vi "ScaleRawData.vi"(4 "Vx,Vy,Vsum as signals or\ntrue X,Y,Z signal (1,default)":bool=TRUE, 5 "error in (no error)":errorcluster, 6 "All DAQ channels":T3, 7 "Scale Option":i32(ring)=2 items=["ScaleButDoNotCalculatePsi", "CalculatePsi, ButDoNotCompensate", "CompensationAllSignalsByCalcuatedPsi", "DoNotScale(ReadRawVoltageSignals)"], 8 "Params in":T8={"Manual Control"={"Rotation Control"={"Phase"=0.0, "A amp (0-120)"=75.0, "B amp (0-120)"=53.3, "mean freq  [MHz]\ndefault 39.99"=40.0, "freq difference [Hz]"=2.0, "Enable A"=TRUE, "Enable B"=TRUE}, "X piezo\n [nm]"=0.0, "Y peizo\n [nm]"=0.0, "-Z piezo\n [nm]"=5.012658227848101, "AOM0 \nPower"=0.2}, "Piezo Calibr"={"Px2Vx(AO)"=nan, "Py2Vy(AO)"=nan, "Pz2Vz(AO)"=nan, "Min Px"=nan, "Min Py"=nan, "Min Pz"=nan, "Max Px"=nan, "Max Py"=nan, "Max Pz"=nan}, "Instrument Calibr"={"TQGT"=[], "TetherCenter"={"TrapX_AO 0 [nm]"=nan, "TrapY_AO 0 [nm]"=nan, "TrapZ_AO 0 [nm]"=nan}, "XYZsignal baseline"={"Xsignal0"=nan, "Ysignal0"=nan, "Zsignal0"=nan, "Zsig slope"=nan, "Z bead0"=nan}, "S and P to Vs0"={"Vs0/P"=1.0, "Vs0/S"=1.0}, "Psi"=0.0, "ePS:eRL drift correlation"={"Interc P"=nan, "Slope P"=nan, "Interc S"=nan, "Slope S"=nan}, "Current piezo volt AO"={"Vpx_AO [V]"=nan, "Vpy_AO [V]"=nan, "Vpz_AO [V]"=nan}}, "Cylinder Calibr"={"ZStiff"=nan, "Zsens"=nan, "AngStiff"=nan, "XStiff"=nan, "Xsens"=nan, "MaxEllip"=nan, "YStiff"=nan, "Ysens"=nan, "FocalShift"=nan, "Sfz"=nan, "1/Sz"=nan, "Stau"=nan, "Sfx"=nan, "1/Sx"=nan, "1/Sang"=nan, "Sfy"=nan, "1/Sy"=nan, "1/focal"=nan}, "DAQParams"={"Buffer size"=nan, "Scanning rate"=nan, "Average"=nan, "Sampling rate"=nan, "set dt"=nan}, "DAQ channel offsets"={"A0 [V]"=0.0, "D0 [V]"=0.0, "P0  [V]"=0.0, "S0 [V]"=0.0, "L0 [V]"=0.0, "R0 [V]"=0.0, "Vpx0 [V]"=0.0, "Vpy0 [V]"=0.0, "Vpz0 [V]"=0.0, "Vsum0 [V]"=0.0, "Vpx_AO0 [V]"=0.0, "Vpy_AO0 [V]"=0.0, "Vpz_AO0 [V]"=0.0}, "Z bead polynomial coeffs"=[nan, nan, nan, nan], "Skip button ref"=refnum, "z bead lookup table"={"z signal"=[], "z bead"=[]}, "SP->power Matrix"=[], "Ms2p"=[], "Mp2s"=[], "task in"="Oscilloscope2"} {"Instrument Calibr"."Psi" format="%#_2f"; "Manual Control"."Y peizo\n [nm]" scale=0.0..7000.0; "Manual Control"."AOM0 \nPower" scale=0.0..1.0; "Manual Control"."X piezo\n [nm]" scale=0.0..7000.0; "Manual Control"."Rotation Control"."freq difference [Hz]" step=0.5; "Manual Control"."Rotation Control"."mean freq  [MHz]\ndefault 39.99" min=0.0 step=0.01; "Manual Control"."Rotation Control"."B amp (0-120)" min=0.0 max=120.0 step=0.1; "Manual Control"."Rotation Control"."A amp (0-120)" min=0.0 max=120.0 step=0.1; "Manual Control"."Rotation Control"."Phase" scale=0.0..360.0; "Manual Control"."-Z piezo\n [nm]" scale=1000.0..7000.0}) -> (0 "error out":errorcluster, 1 "Scaled data":T7, 2 "All DAQ channels out":T3, 3 "Params out":T8={"Manual Control"={"Rotation Control"={"Phase"=0.0, "A amp (0-120)"=75.0, "B amp (0-120)"=53.3, "mean freq  [MHz]\ndefault 39.99"=40.0, "freq difference [Hz]"=2.0, "Enable A"=TRUE, "Enable B"=TRUE}, "X piezo\n [nm]"=0.0, "Y peizo\n [nm]"=0.0, "-Z piezo\n [nm]"=5.012658227848101, "AOM0 \nPower"=0.2}, "Piezo Calibr"={"Px2Vx(AO)"=nan, "Py2Vy(AO)"=nan, "Pz2Vz(AO)"=nan, "Min Px"=nan, "Min Py"=nan, "Min Pz"=nan, "Max Px"=nan, "Max Py"=nan, "Max Pz"=nan}, "Instrument Calibr"={"TQGT"=[], "TetherCenter"={"TrapX_AO 0 [nm]"=nan, "TrapY_AO 0 [nm]"=nan, "TrapZ_AO 0 [nm]"=nan}, "XYZsignal baseline"={"Xsignal0"=nan, "Ysignal0"=nan, "Zsignal0"=nan, "Zsig slope"=nan, "Z bead0"=nan}, "S and P to Vs0"={"Vs0/P"=1.0, "Vs0/S"=1.0}, "Psi"=0.0, "ePS:eRL drift correlation"={"Interc P"=nan, "Slope P"=nan, "Interc S"=nan, "Slope S"=nan}, "Current piezo volt AO"={"Vpx_AO [V]"=nan, "Vpy_AO [V]"=nan, "Vpz_AO [V]"=nan}}, "Cylinder Calibr"={"ZStiff"=nan, "Zsens"=nan, "AngStiff"=nan, "XStiff"=nan, "Xsens"=nan, "MaxEllip"=nan, "YStiff"=nan, "Ysens"=nan, "FocalShift"=nan, "Sfz"=nan, "1/Sz"=nan, "Stau"=nan, "Sfx"=nan, "1/Sx"=nan, "1/Sang"=nan, "Sfy"=nan, "1/Sy"=nan, "1/focal"=nan}, "DAQParams"={"Buffer size"=nan, "Scanning rate"=nan, "Average"=nan, "Sampling rate"=nan, "set dt"=nan}, "DAQ channel offsets"={"A0 [V]"=0.0, "D0 [V]"=0.0, "P0  [V]"=0.0, "S0 [V]"=0.0, "L0 [V]"=0.0, "R0 [V]"=0.0, "Vpx0 [V]"=0.0, "Vpy0 [V]"=0.0, "Vpz0 [V]"=0.0, "Vsum0 [V]"=0.0, "Vpx_AO0 [V]"=0.0, "Vpy_AO0 [V]"=0.0, "Vpz_AO0 [V]"=0.0}, "Z bead polynomial coeffs"=[nan, nan, nan, nan], "Skip button ref"=refnum, "z bead lookup table"={"z signal"=[], "z bead"=[]}, "SP->power Matrix"=[], "Ms2p"=[], "Mp2s"=[], "task in"="Oscilloscope2"} {"Instrument Calibr"."Psi" format="%#_2f"; "Manual Control"."Y peizo\n [nm]" scale=0.0..7000.0; "Manual Control"."AOM0 \nPower" scale=0.0..1.0; "Manual Control"."X piezo\n [nm]" scale=0.0..7000.0; "Manual Control"."Rotation Control"."freq difference [Hz]" step=0.5; "Manual Control"."Rotation Control"."mean freq  [MHz]\ndefault 39.99" min=0.0 step=0.01; "Manual Control"."Rotation Control"."B amp (0-120)" min=0.0 max=120.0 step=0.1; "Manual Control"."Rotation Control"."A amp (0-120)" min=0.0 max=120.0 step=0.1; "Manual Control"."Rotation Control"."Phase" scale=0.0..360.0; "Manual Control"."-Z piezo\n [nm]" scale=1000.0..7000.0})   [LabVIEW 2017, in "SignalConverson.lvlib"]
uses:
  SignalConverson.lvlib
  <vilib>/Analysis/NI_AALBase.lvlib
  <vilib>/Analysis/baseanly.llb/A x Vector.vi
  Angle compensated data.ctl
  XYZ Signals.ctl
  Measrured TrapXYZ.ctl
  Set TrapXYZ.ctl
  Data Before Angle Compensation.ctl
  Initialization/Param.ctl
  Initialization/ManualCtrl.ctl
  Initialization/Initialization.lvlib
  Initialization/CylinderCalibrNew.ctl
  <vilib>/Analysis/Matrix/Datatypes/RealMatrix.ctl
  <vilib>/Analysis/Matrix/NI_Matrix.lvlib
  DAQChannelRawData.ctl
  DAQChannelOffsets.ctl
  ScaledData.ctl
panel:
  out "Data before TCT":T1
  out "set TrapXYZ":T2
  out "Measured Piezo Position":T4
  out "X,Y,Z signal":T5
  out "Data after TCT":T6
  out "Data Before TCT":T1
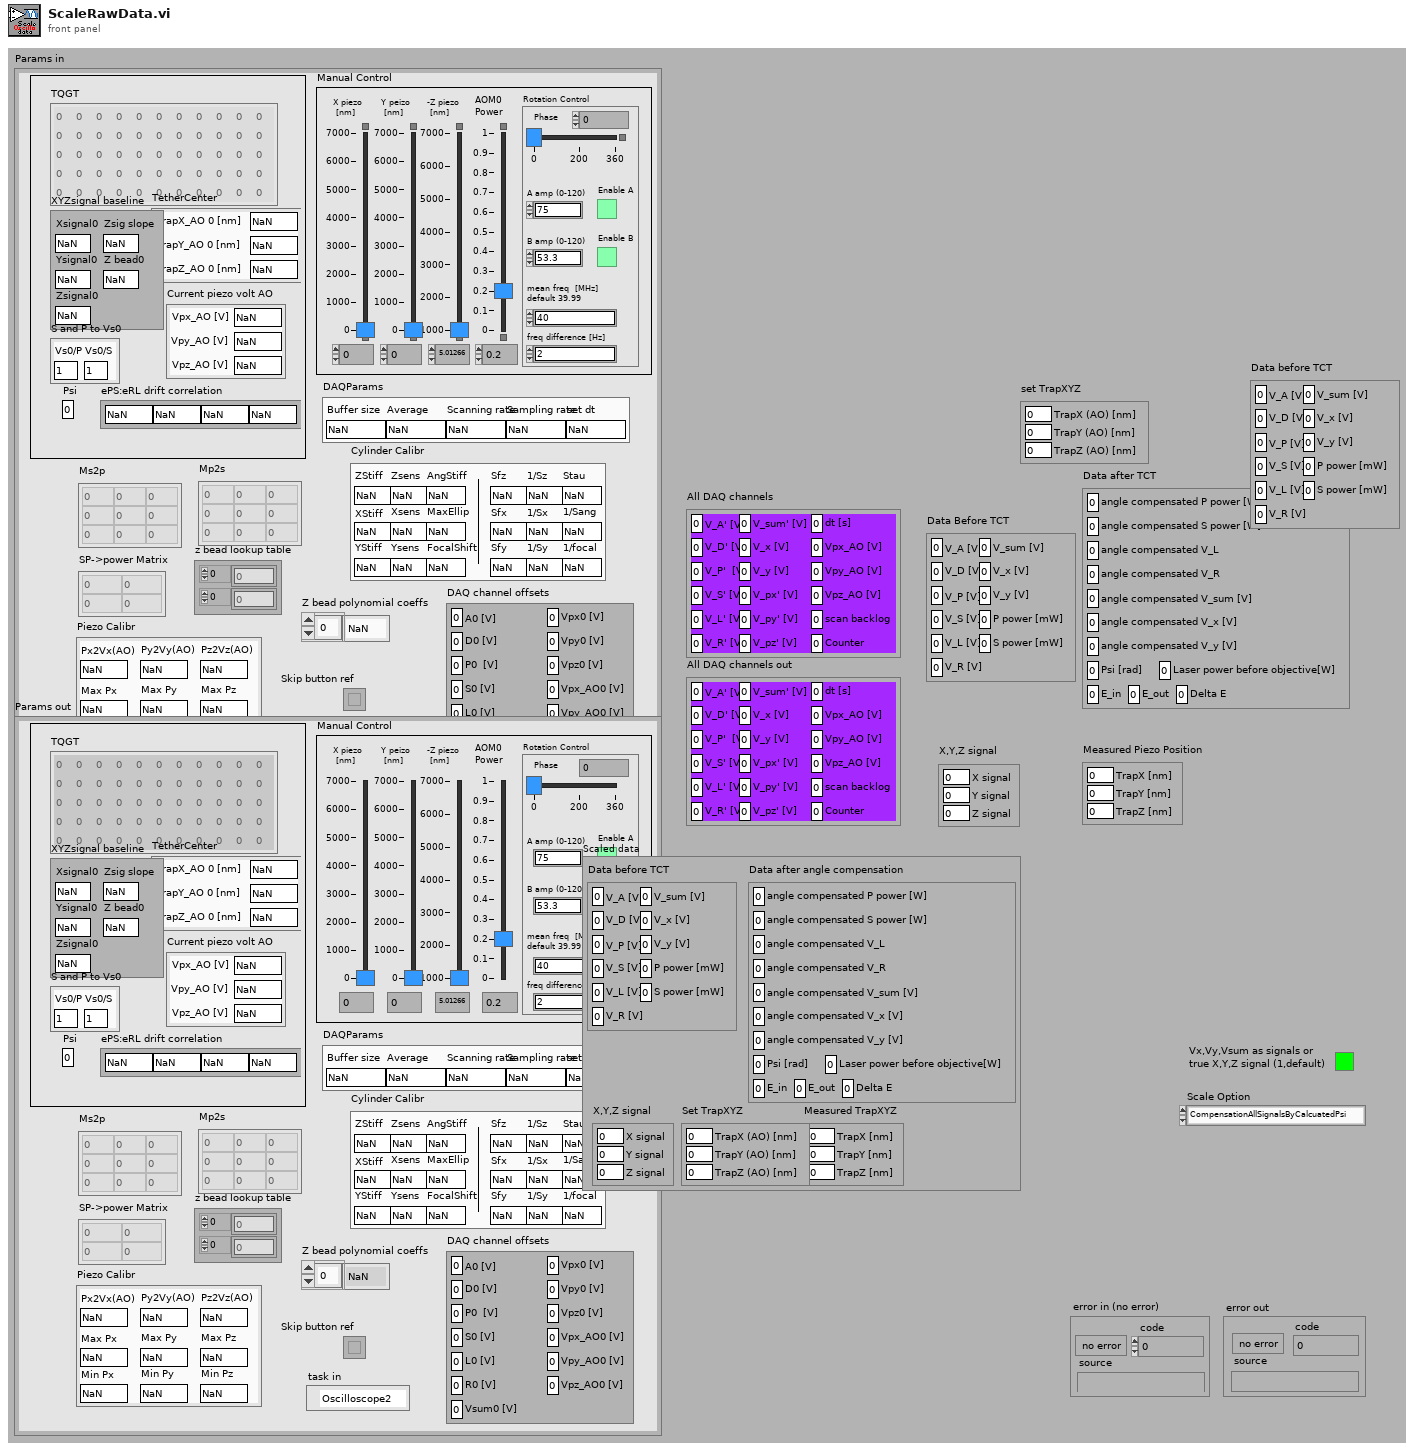
[diagram p1: front panel]
types:
  T1 = typedef "SignalConverson.lvlib/Data Before Angle Compensation.ctl" = cluster{"V_A [V]":dbl, "V_D [V]":dbl, "V_P [V]":dbl, "V_S [V]":dbl, "V_L [V]":dbl, "V_R [V]":dbl, "V_sum [V]":dbl, "V_x [V]":dbl, "V_y [V]":dbl, "P power [mW]":dbl, "S power [mW]":dbl}
  T2 = typedef "SignalConverson.lvlib/Set TrapXYZ.ctl" = cluster{"TrapX (AO) [nm]":dbl, "TrapY (AO) [nm]":dbl, "TrapZ (AO) [nm]":dbl}
  T3 = typedef "SignalConverson.lvlib/DAQChannelRawData.ctl" = cluster{"V_A' [V]":dbl, "V_D' [V]":dbl, "V_P'  [V]":dbl, "V_S' [V]":dbl, "V_L' [V]":dbl, "V_R' [V]":dbl, "V_sum' [V]":dbl, "V_x [V]":dbl, "V_y [V]":dbl, "V_px' [V]":dbl, "V_py' [V]":dbl, "V_pz' [V]":dbl, "dt [s]":dbl, "Vpx_AO [V]":dbl, "Vpy_AO [V]":dbl, "Vpz_AO [V]":dbl, "scan backlog":u32, "Counter":u32}
  T4 = typedef "SignalConverson.lvlib/Measrured TrapXYZ.ctl" = cluster{"TrapX [nm]":dbl, "TrapY [nm]":dbl, "TrapZ [nm]":dbl}
  T5 = typedef "SignalConverson.lvlib/XYZ Signals.ctl" = cluster{"X signal":dbl, "Y signal":dbl, "Z signal":dbl}
  T6 = typedef "SignalConverson.lvlib/Angle compensated data.ctl" = cluster{"angle compensated P power [W]":dbl, "angle compensated S power [W]":dbl, "angle compensated V_L":dbl, "angle compensated V_R":dbl, "angle compensated V_sum [V]":dbl, "angle compensated V_x [V]":dbl, "angle compensated V_y [V]":dbl, "Psi [rad]":dbl, "Laser power before objective[W]":dbl, "E_in":dbl, "E_out":dbl, "Delta E":dbl}
  T7 = typedef "SignalConverson.lvlib/ScaledData.ctl" = cluster{"Measured TrapXYZ":T4, "Data before TCT":T1, "Data after angle compensation":T6, "X,Y,Z signal":T5, "Set TrapXYZ":T2}
  T8 = typedef "Param.ctl" = cluster{"Manual Control":T9, "Piezo Calibr":cluster{"Px2Vx(AO)":dbl, "Py2Vy(AO)":dbl, "Pz2Vz(AO)":dbl, "Min Px":dbl, "Min Py":dbl, "Min Pz":dbl, "Max Px":dbl, "Max Py":dbl, "Max Pz":dbl}, "Instrument Calibr":cluster{"TQGT":dbl[][], "TetherCenter":cluster{"TrapX_AO 0 [nm]":dbl, "TrapY_AO 0 [nm]":dbl, "TrapZ_AO 0 [nm]":dbl}, "XYZsignal baseline":cluster{"Xsignal0":dbl, "Ysignal0":dbl, "Zsignal0":dbl, "Zsig slope":dbl, "Z bead0":dbl}, "S and P to Vs0":cluster{"Vs0/P":dbl, "Vs0/S":dbl}, "Psi":dbl, "ePS:eRL drift correlation":cluster{"Interc P":dbl, "Slope P":dbl, "Interc S":dbl, "Slope S":dbl}, "Current piezo volt AO":cluster{"Vpx_AO [V]":dbl, "Vpy_AO [V]":dbl, "Vpz_AO [V]":dbl}}, "Cylinder Calibr":T10, "DAQParams":cluster{"Buffer size":dbl, "Scanning rate":dbl, "Average":dbl, "Sampling rate":dbl, "set dt":dbl}, "DAQ channel offsets":T11, "Z bead polynomial coeffs":dbl[], "Skip button ref":refnum<vi>, "z bead lookup table":cluster{"z signal":dbl[], "z bead":dbl[]}, "SP->power Matrix":T12, "Ms2p":T12, "Mp2s":T12, "task in":refnum<k21>}
  T9 = typedef "Initialization.lvlib/ManualCtrl.ctl" = cluster{"Rotation Control":cluster{"Phase":dbl, "A amp (0-120)":dbl, "B amp (0-120)":dbl, "mean freq  [MHz]\ndefault 39.99":dbl, "freq difference [Hz]":dbl, "Enable A":bool, "Enable B":bool}, "X piezo\n [nm]":dbl, "Y peizo\n [nm]":dbl, "-Z piezo\n [nm]":dbl, "AOM0 \nPower":dbl}
  T10 = typedef "Initialization.lvlib/CylinderCalibrNew.ctl" = cluster{"ZStiff":dbl, "Zsens":dbl, "AngStiff":dbl, "XStiff":dbl, "Xsens":dbl, "MaxEllip":dbl, "YStiff":dbl, "Ysens":dbl, "FocalShift":dbl, "Sfz":dbl, "1/Sz":dbl, "Stau":dbl, "Sfx":dbl, "1/Sx":dbl, "1/Sang":dbl, "Sfy":dbl, "1/Sy":dbl, "1/focal":dbl}
  T11 = typedef "SignalConverson.lvlib/DAQChannelOffsets.ctl" = cluster{"A0 [V]":dbl, "D0 [V]":dbl, "P0  [V]":dbl, "S0 [V]":dbl, "L0 [V]":dbl, "R0 [V]":dbl, "Vpx0 [V]":dbl, "Vpy0 [V]":dbl, "Vpz0 [V]":dbl, "Vsum0 [V]":dbl, "Vpx_AO0 [V]":dbl, "Vpy_AO0 [V]":dbl, "Vpz_AO0 [V]":dbl}
  T12 = typedef "NI_Matrix.lvlib/RealMatrix.ctl" = dbl[][]
  T13 = cluster{"Px2Vx(AO)":dbl, "Py2Vy(AO)":dbl, "Pz2Vz(AO)":dbl, "Min Px":dbl, "Min Py":dbl, "Min Pz":dbl, "Max Px":dbl, "Max Py":dbl, "Max Pz":dbl}
  T14 = typedef "Initialization.lvlib/New Param_170907.ctl" = cluster{"Manual Control":T9, "Piezo Calibr":cluster{"Px2Vx(AO)":dbl, "Py2Vy(AO)":dbl, "Pz2Vz(AO)":dbl, "Min Px":dbl, "Min Py":dbl, "Min Pz":dbl, "Max Px":dbl, "Max Py":dbl, "Max Pz":dbl, "Vx0 (V)":dbl, "Vy0 (V)":dbl, "Vz0 (V)":dbl}, "Instrument Calibr":cluster{"Angular compensation coeffs":dbl[][], "TetherCenter":cluster{"TrapX_AO 0 [nm]":dbl, "TrapY_AO 0 [nm]":dbl, "TrapZ_AO 0 [nm]":dbl}, "XYZsignal baseline":cluster{"Xsignal0":dbl, "Ysignal0":dbl, "Zsignal0":dbl, "Zsig slope":dbl, "Z bead0":dbl}, "S and P to Vs0":cluster{"Vs0/P":dbl, "Vs0/S":dbl}, "Psi":dbl, "ePS:eRL drift correlation":cluster{"Interc P":dbl, "Slope P":dbl, "Interc S":dbl, "Slope S":dbl}, "Current piezo volt AO":cluster{"Vpx_AO [V]":dbl, "Vpy_AO [V]":dbl, "Vpz_AO [V]":dbl}}, "Cylinder Calibr":T10, "DAQParams":cluster{"Buffer size":dbl, "Scanning rate":dbl, "Average":dbl, "Sampling rate":dbl, "set dt":dbl}, "DAQ channel offsets":T11, "Z bead polynomial coeffs":dbl[], "Skip button ref":refnum<vi>, "z bead lookup table":cluster{"z signal":dbl[], "z bead":dbl[]}, "SP->power Matrix":T12, "Ms2p":T12, "Mp2s":T12, "Polynomial coeff V_px,y,z 2 position (nm)":dbl[][], "task in":refnum<k21>}
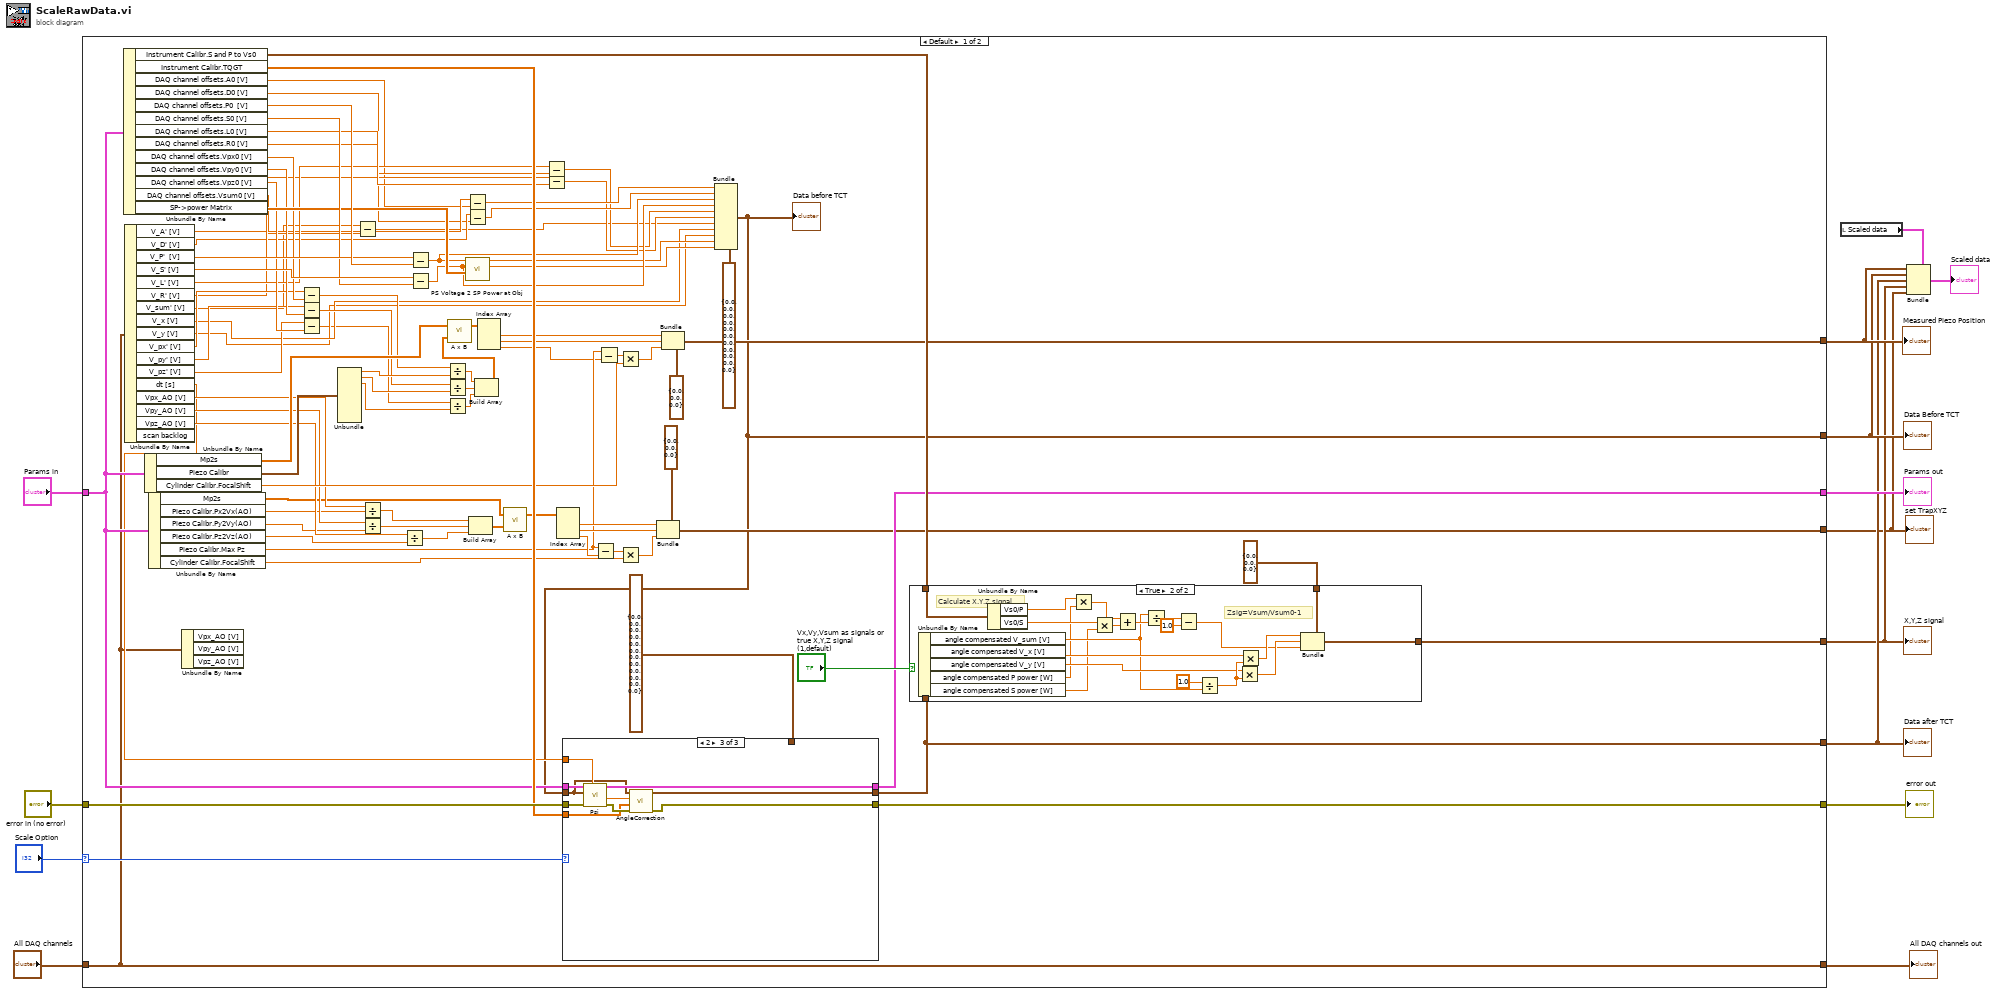
[diagram p0: block diagram]
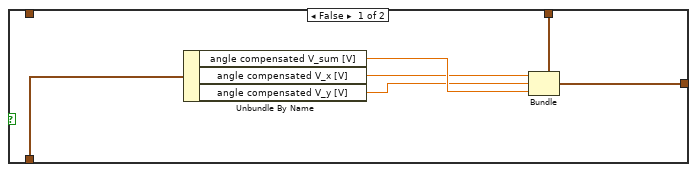
[diagram p2: hidden frame]
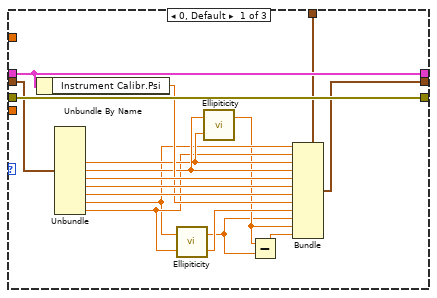
[diagram p3: hidden frame]
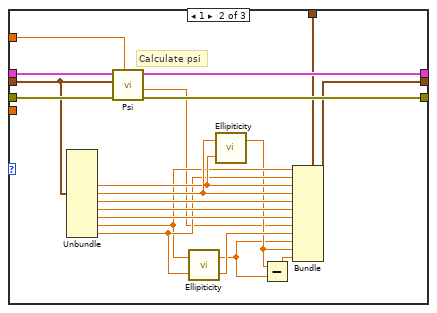
[diagram p4: hidden frame]
diagram:
  n1 = case shown="Default" "Scale Option" {
    selector: "Scale Option" -> [w101 _]
    tunnel: "All DAQ channels" -> [w34 w179]
    tunnel: "Params in" -> [w70 w180]
    tunnel: "error in (no error)" -> [w104 w181]
    tunnel: [w102 w181] -> w2
    tunnel: [w98 w180] -> w13
    tunnel: [w40 _] -> w4
    tunnel: [w39 _] -> w5
    tunnel: [w24 _] -> w6
    tunnel: [w35 _] -> w7
    tunnel: [w34 w179] -> w9
    tunnel: [w25 _] -> w3
    frame Default {
      n2 = Unbundle By Name(w70) -> ("Instrument Calibr.S and P to Vs0"=w100:cluster{"Vs0/P":dbl, "Vs0/S":dbl}, "Instrument Calibr.TQGT"=w103:dbl[][], "DAQ channel offsets.A0 [V]"=w55:dbl, "DAQ channel offsets.D0 [V]"=w54:dbl, "DAQ channel offsets.P0  [V]"=w97:dbl, "DAQ channel offsets.S0 [V]"=w94:dbl, "DAQ channel offsets.L0 [V]"=w68:dbl, "DAQ channel offsets.R0 [V]"=w69:dbl, "DAQ channel offsets.Vpx0 [V]"=w81:dbl, "DAQ channel offsets.Vpy0 [V]"=w80:dbl, "DAQ channel offsets.Vpz0 [V]"=w79:dbl, "DAQ channel offsets.Vsum0 [V]"=w22:dbl, "SP->power Matrix"=w93:T12)
      n3 = Unbundle By Name(w34) -> ("V_A' [V]"=w57:dbl, "V_D' [V]"=w56:dbl, "V_P'  [V]"=w96:dbl, "V_S' [V]"=w95:dbl, "V_L' [V]"=w67:dbl, "V_R' [V]"=w66:dbl, "V_sum' [V]"=w21:dbl, "V_x [V]"=w45:dbl, "V_y [V]"=w44:dbl, "V_px' [V]"=w78:dbl, "V_py' [V]"=w77:dbl, "V_pz' [V]"=w76:dbl, "dt [s]"=w43:dbl, "Vpx_AO [V]"=w73:dbl, "Vpy_AO [V]"=w72:dbl, "Vpz_AO [V]"=w71:dbl)  [unwired: 1 out]
      n4 = Unbundle By Name(w70) -> ("Mp2s"=w82:T12, "Piezo Calibr"=w84:T13, "Cylinder Calibr.FocalShift"=w83:dbl)
      n5 = Unbundle By Name(w70) -> ("Mp2s"=w59:T12, "Piezo Calibr.Px2Vx(AO)"=w65:dbl, "Piezo Calibr.Py2Vy(AO)"=w64:dbl, "Piezo Calibr.Pz2Vz(AO)"=w63:dbl, "Piezo Calibr.Max Pz"=w19:dbl, "Cylinder Calibr.FocalShift"=w30:dbl)
      n6 = Unbundle By Name(w34) -> ()  [unwired: 3 out]
      n7 = Subtract(x=w78, y=w81) -> (x-y=w75:dbl)
      n8 = Subtract(x=w77, y=w80) -> (x-y=w74:dbl)
      n9 = Subtract(x=w76, y=w79) -> (x-y=w18:dbl)
      n10 = Unbundle(w84) -> ("Px2Vx(AO)"=w87:dbl, "Py2Vy(AO)"=w88:dbl, "Pz2Vz(AO)"=w89:dbl)  [unwired: 6 out]
      n11 = Subtract(x=w21, y=w22) -> (x-y=w20:dbl)
      n12 = Divide(x=w73, y=w65) -> (x/y=w61:dbl)
      n13 = Divide(x=w72, y=w64) -> (x/y=w62:dbl)
      n14 = Divide(x=w71, y=w63) -> (x/y=w33:dbl)
      n15 = Subtract(x=w96, y=w97) -> (x-y=w51:dbl)
      n16 = Subtract(x=w95, y=w94) -> (x-y=w50:dbl)
      n17 = Divide(x=w75, y=w87) -> (x/y=w90:dbl)
      n18 = Divide(x=w74, y=w88) -> (x/y=w91:dbl)
      n19 = Divide(x=w18, y=w89) -> (x/y=w92:dbl)
      n20 = Subtract(x=w57, y=w55) -> (x-y=w53:dbl)
      n21 = Subtract(x=w56, y=w54) -> (x-y=w52:dbl)
      n22 = call "PS Voltage 2 SP Power at Obj.vi"("SP -> Power Matrix"=w93, "Volts S"=w50, "Volts P"=w51) -> ("Power S"=w46:dbl, "Power P"=w47:dbl)  [unwired: 3 in]
      n23 = Build Array(w61, w62, w33) -> (w60:dbl[])
      n24 = Build Array(w90, w91, w92) -> (w85:dbl[])
      n25 = call-poly <vilib>:"A x B.vi"("Vector"=w85, "A"=w82) -> ("A x Vector"=w86:dbl[])  [unwired: 1 out]
      n26 = Index Array(array=w86) -> (element #1=w37:dbl, element #2=w36:dbl, element #3=w17:dbl)  [unwired: 3 in]
      n27 = call-poly <vilib>:"A x B.vi"("Vector"=w60, "A"=w59) -> ("A x Vector"=w58:dbl[])  [unwired: 1 out]
      n28 = Subtract(x=w67, y=w68) -> (x-y=w49:dbl)
      n29 = Subtract(x=w66, y=w69) -> (x-y=w48:dbl)
      n30 = Index Array(array=w58) -> (element #1=w29:dbl, element #2=w28:dbl, element #3=w32:dbl)  [unwired: 3 in]
      n31 = Subtract(x=w19, y=w32) -> (x-y=w31:dbl)
      n32 = Subtract(x=w19, y=w17) -> (x-y=w16:dbl)
      n33 = Multiply(x=w31, y=w30) -> (x*y=w27:dbl)
      n34 = Multiply(x=w16, y=w83) -> (x*y=w15:dbl)
      n35 = Bundle(cluster=T2 {"TrapX (AO) [nm]"=0.0, "TrapY (AO) [nm]"=0.0, "TrapZ (AO) [nm]"=0.0} ("set TrapXYZ"), "TrapX (AO) [nm]"=w29, "TrapY (AO) [nm]"=w28, "TrapZ (AO) [nm]"=w27) -> (w25:T2)
      n36 = Bundle(cluster=T4 {"TrapX [nm]"=0.0, "TrapY [nm]"=0.0, "TrapZ [nm]"=0.0} ("Measured Piezo Position"), "TrapX [nm]"=w37, "TrapY [nm]"=w36, "TrapZ [nm]"=w15) -> (w35:T4)
      n37 = Bundle(cluster=T1 {"V_A [V]"=0.0, "V_D [V]"=0.0, "V_P [V]"=0.0, "V_S [V]"=0.0, "V_L [V]"=0.0, "V_R [V]"=0.0, "V_sum [V]"=0.0, "V_x [V]"=0.0, "V_y [V]"=0.0, "P power [mW]"=0.0, "S power [mW]"=0.0} ("Data before TCT"), "V_A [V]"=w53, "V_D [V]"=w52, "V_P [V]"=w51, "V_S [V]"=w50, "V_L [V]"=w49, "V_R [V]"=w48, "V_sum [V]"=w20, "V_x [V]"=w45, "V_y [V]"=w44, "P power [mW]"=w47, "S power [mW]"=w46) -> (w24:T1)
      "Data before TCT" <- w24
      n38 = case shown="2" w101 {
        tunnel: w104 -> [w148 w167 w177]
        tunnel: [w140 w150 w170] -> w39
        tunnel: [w148 w168 w176] -> w102
        tunnel: w103 -> [_ _ w175]
        tunnel: w70 -> [w147 w166 w174]
        tunnel: [w147 w165 w173] -> w98
        tunnel: w24 -> [w146 w152 w169]
        tunnel: w43 -> [_ w164 w171]
        tunnel: T6 {"angle compensated P power [W]"=0.0, "angle compensated S power [W]"=0.0, "angle compensated V_L"=0.0, "angle compensated V_R"=0.0, "angle compensated V_sum [V]"=0.0, "angle compensated V_x [V]"=0.0, "angle compensated V_y [V]"=0.0, "Psi [rad]"=0.0, "Laser power before objective[W]"=0.0, "E_in"=0.0, "E_out"=0.0, "Delta E"=0.0} ("Data after TCT") -> [w145 w151 _]
        frame 0, Default {
          n39 = Unbundle By Name(w147) -> ("Instrument Calibr.Psi"=w141:dbl)
          n40 = Unbundle(w146) -> ("V_L [V]"=w138:dbl, "V_R [V]"=w139:dbl, "V_sum [V]"=w144:dbl, "V_x [V]"=w143:dbl, "V_y [V]"=w142:dbl, "P power [mW]"=w136:dbl, "S power [mW]"=w137:dbl)  [unwired: 4 out]
          n41 = call "Ellipiticity.vi"("S"=w137, "P"=w136) -> ("P+S"=w135:dbl, "(P-S)/(P+S)"=w133:dbl)
          n42 = call "Ellipiticity.vi"("S"=w138, "P"=w139) -> ("(P-S)/(P+S)"=w134:dbl)  [unwired: 1 out]
          n43 = Subtract(x=w134, y=w133) -> (x-y=w132:dbl)
          n44 = Bundle(cluster=w145, "angle compensated P power [W]"=w136, "angle compensated S power [W]"=w137, "angle compensated V_L"=w138, "angle compensated V_R"=w139, "angle compensated V_sum [V]"=w144, "angle compensated V_x [V]"=w143, "angle compensated V_y [V]"=w142, "Psi [rad]"=w141, "Laser power before objective[W]"=w135, "E_in"=w133, "E_out"=w134, "Delta E"=w132) -> (w140:T6)
        }
        frame 1 {
          # "Calculate psi"
          n45 = Unbundle(w152) -> ("V_L [V]"=w159:dbl, "V_R [V]"=w160:dbl, "V_sum [V]"=w163:dbl, "V_x [V]"=w162:dbl, "V_y [V]"=w161:dbl, "P power [mW]"=w157:dbl, "S power [mW]"=w158:dbl)  [unwired: 4 out]
          n46 = call "Psi.vi"("dt [s]"=w164, "error in (no error)"=w167, "Data before TCT"=w152, "Params in"=w166) -> ("error out"=w168:errorcluster, "Psi"=w149:dbl, "Params out"=w165:T14)  [unwired: 2 in]
          n47 = call "Ellipiticity.vi"("S"=w158, "P"=w157) -> ("P+S"=w156:dbl, "(P-S)/(P+S)"=w154:dbl)
          n48 = call "Ellipiticity.vi"("S"=w159, "P"=w160) -> ("(P-S)/(P+S)"=w155:dbl)  [unwired: 1 out]
          n49 = Subtract(x=w155, y=w154) -> (x-y=w153:dbl)
          n50 = Bundle(cluster=w151, "angle compensated P power [W]"=w157, "angle compensated S power [W]"=w158, "angle compensated V_L"=w159, "angle compensated V_R"=w160, "angle compensated V_sum [V]"=w163, "angle compensated V_x [V]"=w162, "angle compensated V_y [V]"=w161, "Psi [rad]"=w149, "Laser power before objective[W]"=w156, "E_in"=w154, "E_out"=w155, "Delta E"=w153) -> (w150:T6)
        }
        frame 2 {
          n51 = call "Psi.vi"("dt [s]"=w171, "error in (no error)"=w177, "Data before TCT"=w169, "Params in"=w174) -> ("error out"=w178:errorcluster, "Psi"=w172:dbl, "Params out"=w173:T14)  [unwired: 2 in]
          n52 = call "AngleCorrection.vi"("error in (no error)"=w178, "TQGT"=w175, "Psi"=w172, "Data Before TCT"=w169) -> ("error out"=w176:errorcluster, "Data after TCT"=w170:T6)  [unwired: 2 in]
        }
      }
      n53 = case shown="True" "Vx,Vy,Vsum as signals or\ntrue X,Y,Z signal (1,default)" {
        tunnel: w100 -> [_ w124]
        tunnel: [w109 w112] -> w40
        tunnel: w39 -> [w108 w121]
        tunnel: T5 {"X signal"=0.0, "Y signal"=0.0, "Z signal"=0.0} ("X,Y,Z signal") -> [w110 w111]
        frame False {
          n54 = Unbundle By Name(w108) -> ("angle compensated V_sum [V]"=w107:dbl, "angle compensated V_x [V]"=w106:dbl, "angle compensated V_y [V]"=w105:dbl)
          n55 = Bundle(cluster=w110, "X signal"=w106, "Y signal"=w105, "Z signal"=w107) -> (w109:T5)
        }
        frame True {
          # "Zsig=Vsum/Vsum0-1"
          # "Calculate X.Y.Z signal"
          n56 = Unbundle By Name(w121) -> ("angle compensated V_sum [V]"=w118:dbl, "angle compensated V_x [V]"=w120:dbl, "angle compensated V_y [V]"=w119:dbl, "angle compensated P power [W]"=w117:dbl, "angle compensated S power [W]"=w116:dbl)
          n57 = Unbundle By Name(w124) -> ("Vs0/P"=w127:dbl, "Vs0/S"=w128:dbl)
          n58 = Multiply(x=w127, y=w117) -> (x*y=w130:dbl)
          n59 = Multiply(x=w128, y=w116) -> (x*y=w129:dbl)
          n60 = Add(x=w130, y=w129) -> (x+y=w131:dbl)
          n61 = Divide(x=w118, y=w131) -> (x/y=w123:dbl)
          n62 = Subtract(x=w123, y=1.0 ("x")) -> (x-y=w113:dbl)
          n63 = Divide(x=1.0, y=w118) -> (x/y=w126:dbl)
          n64 = Multiply(x=w119, y=w126) -> (x*y=w114:dbl)
          n65 = Multiply(x=w120, y=w126) -> (x*y=w115:dbl)
          n66 = Bundle(cluster=w111, "X signal"=w115, "Y signal"=w114, "Z signal"=w113) -> (w112:T5)
        }
      }
    }
    frame 3 {
    }
  }
  "Params out" <- w13
  "X,Y,Z signal" <- w4
  "Data after TCT" <- w5
  "Data Before TCT" <- w6
  "Measured Piezo Position" <- w7
  "All DAQ channels out" <- w9
  "set TrapXYZ" <- w3
  "error out" <- w2
  n67 = local read "Scaled data"() -> (w8:T7)
  n68 = Bundle(cluster=w8, "Measured TrapXYZ"=w7, "Data before TCT"=w6, "Data after angle compensation"=w5, "X,Y,Z signal"=w4, "Set TrapXYZ"=w3) -> (→"Scaled data":T7)
